vi "Untitled 3 (SubVI).vi"(10 "Array in":i32[][](array[numeric]), 11 "Memory in":u8) -> (2 "Boolean":bool, 3 "Memory out":u8)   [LabVIEW 2020]
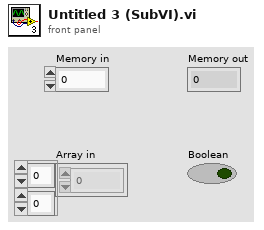
[diagram p1: front panel]
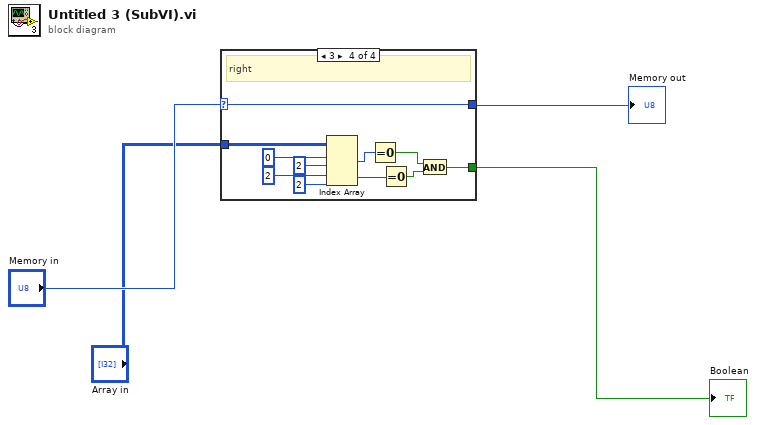
[diagram p0: block diagram]
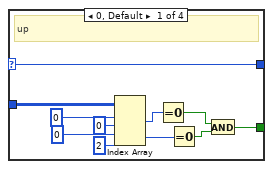
[diagram p2: hidden frame]
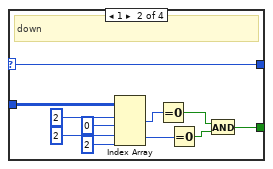
[diagram p3: hidden frame]
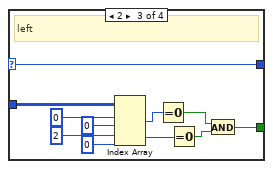
[diagram p4: hidden frame]
diagram:
  n1 = case shown="3" "Memory in" {
    selector: "Memory in" -> [w6 w17 w28 w39]
    tunnel: "Array in" -> [w15 w26 w37 w48]
    tunnel: [w7 w18 w29 w40] -> w3
    tunnel: [w6 w17 w28 w39] -> w2
    frame 0, Default {
      # "up"
      n2 = Index Array(array=w15, index (row) #1=0 ("index (row)"), index (col) #1=0 ("disabled index (col)"), index (row) #2=0 ("disabled index (row)"), index (col) #2=2 ("disabled index (col)")) -> (element #1=w11:i32, element #2=w10:i32)
      n3 = Equal To 0?(x=w11) -> (x = 0?=w8:bool)
      n4 = Equal To 0?(x=w10) -> (x = 0?=w9:bool)
      n5 = And(x=w8, y=w9) -> (x .and. y?=w7:bool)
    }
    frame 1 {
      # "down"
      n6 = Index Array(array=w26, index (row) #1=2 ("index (row)"), index (col) #1=0 ("disabled index (col)"), index (row) #2=2 ("disabled index (row)"), index (col) #2=2 ("disabled index (col)")) -> (element #1=w22:i32, element #2=w21:i32)
      n7 = Equal To 0?(x=w22) -> (x = 0?=w19:bool)
      n8 = Equal To 0?(x=w21) -> (x = 0?=w20:bool)
      n9 = And(x=w19, y=w20) -> (x .and. y?=w18:bool)
    }
    frame 2 {
      # "left"
      n10 = Index Array(array=w37, index (row) #1=0 ("index (row)"), index (col) #1=0 ("disabled index (col)"), index (row) #2=2 ("disabled index (row)"), index (col) #2=0 ("disabled index (col)")) -> (element #1=w33:i32, element #2=w32:i32)
      n11 = Equal To 0?(x=w33) -> (x = 0?=w30:bool)
      n12 = Equal To 0?(x=w32) -> (x = 0?=w31:bool)
      n13 = And(x=w30, y=w31) -> (x .and. y?=w29:bool)
    }
    frame 3 {
      # "right"
      n14 = Index Array(array=w48, index (row) #1=0 ("index (row)"), index (col) #1=2 ("disabled index (col)"), index (row) #2=2 ("disabled index (row)"), index (col) #2=2 ("disabled index (col)")) -> (element #1=w44:i32, element #2=w43:i32)
      n15 = Equal To 0?(x=w44) -> (x = 0?=w41:bool)
      n16 = Equal To 0?(x=w43) -> (x = 0?=w42:bool)
      n17 = And(x=w41, y=w42) -> (x .and. y?=w40:bool)
    }
  }
  "Boolean" <- w3
  "Memory out" <- w2
